vi "Read Screen Tap Position.vi"   [LabVIEW 2011, in "LVH-Leap.lvlib"]
doc: "Read screen tap gesture position. Use the polymorphic instance to select between one screen tap and N screen tap gestures."
uses:
  LVH-Leap.lvlib
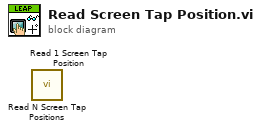
[diagram p0: block diagram]
diagram:
  n1 = call "Read N Screen Tap Positions.vi"() -> ()  [unwired: 8 in, 4 out]
  n2 = call "Read 1 Screen Tap Position.vi"() -> ()  [unwired: 8 in, 4 out]
